vi "加表当量.vi"(11 "x":dbl) -> (3 "子数组":u8[](array[numeric]))   [LabVIEW 2012]
panel:
  out "最接近的整数值":dbl
  out "*(类型 *) &x":u8[](array[numeric])
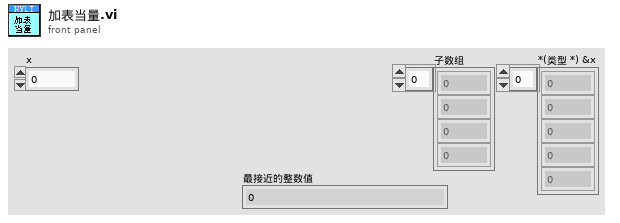
[diagram p1: front panel]
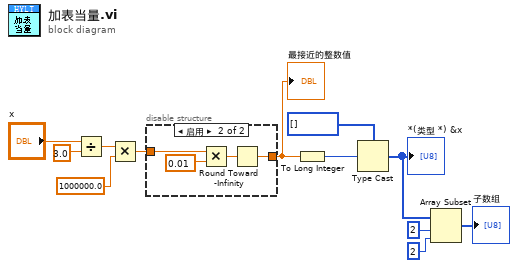
[diagram p0: block diagram]
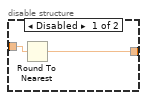
[diagram p2: hidden frame]
diagram:
  n1 = Divide(x="x", y=3.0) -> (x/y=w11:dbl)
  n2 = Multiply(x=w11, y=1000000.0) -> (x*y=w10:dbl)
  n3 = disable-structure shown="启用" {
    disable-tunnel: w10 -> [w14 w17]
    disable-tunnel: [w13 w18] -> w9
    frame Disabled {
      n4 = Round To Nearest(number=w14) -> (nearest integer value=w13:dbl)
    }
    frame Enabled {
      n5 = Multiply(x=w17, y=0.01) -> (x*y=w16:dbl)
      n6 = Round Toward -Infinity(1:w16) -> (0:w18:dbl)
    }
  }
  "最接近的整数值" <- w9
  n7 = To Long Integer(number=w9) -> (32bit integer=w8:i32)
  n8 = Type Cast(type=u8[] [], x=w8) -> (*(type *) &x=w5:u8[])
  "*(类型 *) &x" <- w5
  n9 = Array Subset(array=w5, index=2 ("索引"), length=2 ("长度")) -> (→"子数组":u8[])
